vi "Decrypt_All_Files_In_Hierarchy.vi"(8 "error in (no error)":errorcluster, 11 "object in":refnum<class "Crypter.lvclass">) -> (0 "error out":errorcluster, 3 "object out":refnum<class "Crypter.lvclass">)   [LabVIEW 2016, in "Crypter.lvclass"]
uses:
  Crypter.lvclass
  Folder_Mgmt/Folder_Mgmt.lvclass
  C:/Users/Marco Preziani/Documents/DOME-LV16/Crypter/Crypter.lvclass
  Crypter.lvclass/Crypter.ctl
  Folder_Mgmt/Folder_Mgmt.lvclass/Folder_Mgmt.ctl
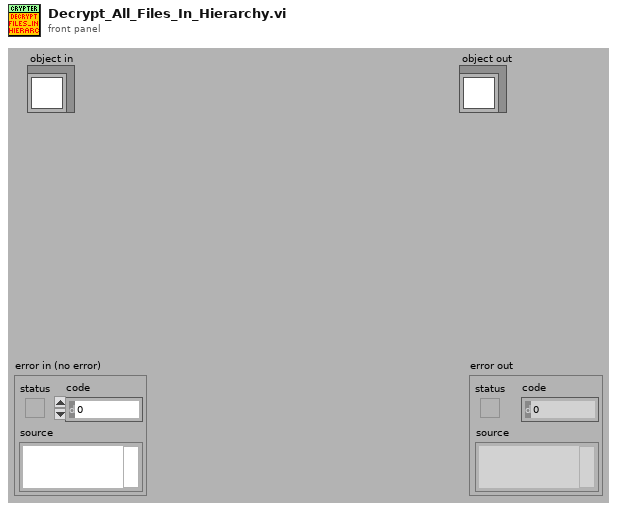
[diagram p1: front panel]
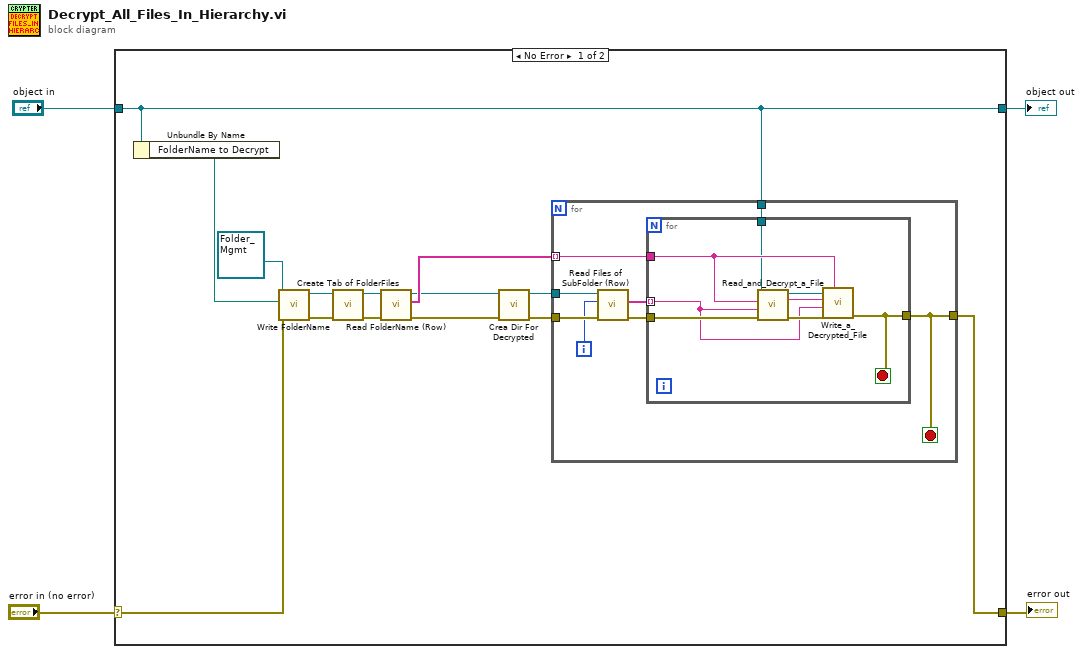
[diagram p0: block diagram]
diagram:
  n1 = case shown="No Error" "error in (no error)" {
    selector: "error in (no error)" -> [w12 w36]
    tunnel: [w11 w36] -> w3
    tunnel: [w13 w35] -> w1
    tunnel: "object in" -> [w13 w35]
    frame No Error {
      n2 = Unbundle By Name(w13) -> ("FolderName to Decrypt"=w15:path)
      n3 = call "Write FolderName.vi"("error in (no error)"=w12, "FolderName"=w15, "Folder_Mgmt in"=refnum<class "Folder_Mgmt.lvclass"> refnum ("Folder_Mgmt.lvclass")) -> ("error out"=w17:errorcluster, "Folder_Mgmt out"=w18:refnum<class "Folder_Mgmt.lvclass">)  [unwired: 7 in]
      n4 = call "Create Tab of FolderFiles.vi"("error in (no error)"=w17, "Folder_Mgmt in"=w18) -> ("error out"=w7:errorcluster, "Folder_Mgmt out"=w8:refnum<class "Folder_Mgmt.lvclass">)  [unwired: 8 in]
      n5 = call "Read FolderName (Row).vi"("error in (no error)"=w7, "Folder_Mgmt in"=w8) -> ("error out"=w6:errorcluster, "FolderName (Row)"=w16:string[], "Folder_Mgmt out"=w5:refnum<class "Folder_Mgmt.lvclass">)  [unwired: 7 in]
      n6 = call "Crea Dir For Decrypted.vi"("error in (no error)"=w6, "Crypter.lvclass"=w5) -> ("error out"=w10:errorcluster, "Crypter.lvclass 2"=w9:refnum<class "Folder_Mgmt.lvclass">)  [unwired: 7 in, 1 out]
      n7 = for {
        tunnel: w9 -> [w26]
        tunnel: w16 -> [w21] mode=indexing
        tunnel: w10 -> [w25]
        tunnel: w13 -> [w20]
        tunnel: [w19] -> w11
        i -> [w23]
        stop <- w19 stop-if-true
        n8 = call "Read Files of SubFolder (Row).vi"("error in (no error)"=w25, "RowIndex"=w23, "Folder_Mgmt in"=w26) -> ("error out"=w24:errorcluster, "FolderFiles (Row)"=w22:string[])  [unwired: 6 in, 1 out]
        n9 = for {
          tunnel: w24 -> [w31]
          tunnel: w21 -> [w29]
          tunnel: w22 -> [w30] mode=indexing
          tunnel: w20 -> [w28]
          tunnel: [w27] -> w19
          stop <- w27 stop-if-true
          n10 = call-dynamic "Read_and_Decrypt_a_File.vi"("error in (no error)"=w31, "name of File"=w30, "name of Folder"=w29, "object in"=w28) -> ("error out"=w32:errorcluster, "Dencrypted text"=w33:string, "object out"=w34:refnum<class "Crypter.lvclass">)  [unwired: 5 in]
          n11 = call-dynamic "Write_a_Decrypted_File.vi"("name of Folder"=w29, "error in (no error)"=w32, "name of file"=w30, "Dencrypted text"=w33, "object in"=w34) -> ("error out"=w27:errorcluster)  [unwired: 5 in, 1 out]
        }
      }
    }
    frame Error {
    }
  }
  "error out" <- w3
  "object out" <- w1
